vi "Main.vi"(10 "JQMHStartup":refnum<class "ModuleStartup.lvclass">, 11 "SingleLoopTemplate in":refnum<class "SingleLoopTemplate.lvclass">) -> ()   [LabVIEW 2024, in "SingleLoopTemplate.lvclass"]
uses:
  SingleLoopTemplate.lvclass
  RQMHCore/ModuleCore/Module.lvclass/Module.ctl
  RQMHCore/ActionStack/Stack/Stack.lvclass/Stack.ctl
  SingleLoopTemplate.lvclass/SingleLoopTemplate.ctl
  C:/Git/JA/JQMH/RQMHCore/ModuleCore/Module.lvclass
  C:/Git/JA/JQMH/ModuleTemplates/SingleLoopTemplate/SingleLoopTemplate.lvclass
  RQMHCore/ModuleCore/Module.lvclass
  RQMHCore/Startup/ModuleStartup.lvclass
  RQMHCore/ModuleCore/Reply.ctl
  <vilib>/Utility/miscctls.llb/LVPointTypeDef.ctl
  RQMHCore/ModuleCore/InitialiseReplyArgs.ctl
  Do Something ReplyArgs.ctl
  RQMHCore/ActionStack/Stack/Stack.lvclass
  RQMHCore/ActionStack/Stack/StackFromSingleWithPayload.vi
  RQMHCore/ActionStack/Stack/InitFromString.vi
  RQMHCore/ActionStack/Stack/AppendStacks.vi
panel:
  out "error out":errorcluster
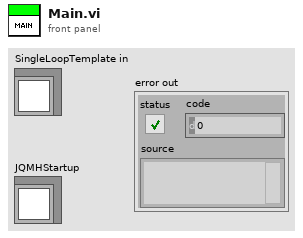
[diagram p1: front panel]
types:
  T1 = typedef "SingleLoopTemplate.lvclass/Request Events--cluster.ctl" = cluster{"Do Something":refnum<user-event>}
  T2 = cluster{"StandardRequests":refnum<event-registration>, "Event Registration Refnum":refnum<event-registration>}
  T3 = cluster{"Module":refnum<class "SingleLoopTemplate.lvclass">, "Args":string}
  T4 = typedef "Module.lvclass/Reply.ctl" = cluster{"Expects Reply":bool, "Reply":refnum<notifier>}
  T5 = enum32{"Invalid", "Standard", "Closed", "Hidden", "Minimized", "Maximized"}
  T6 = typedef "Module.lvclass/InitialiseReplyArgs.ctl" = cluster{"Did Init?":bool}
  T7 = typedef "LVPointTypeDef.ctl" = cluster{"Horizontal":i16, "Vertical":i16}
  T8 = typedef "SingleLoopTemplate.lvclass/Do Something ReplyArgs.ctl" = cluster{"Value":dbl}
  T9 = typedef "JQMHModule.lvclass/Show Front Panel--Args.ctl" = variant
  T10 = typedef "JQMHModule.lvclass/Show Block Diagram.ctl" = bool
  T11 = typedef "JQMHModule.lvclass/Reply.ctl" = cluster{"Expects Reply":bool, "Reply":refnum<notifier>}
  T12 = typedef "SingleLoopTemplate.lvclass/Do Something Args.ctl" = cluster{"Msg":string}
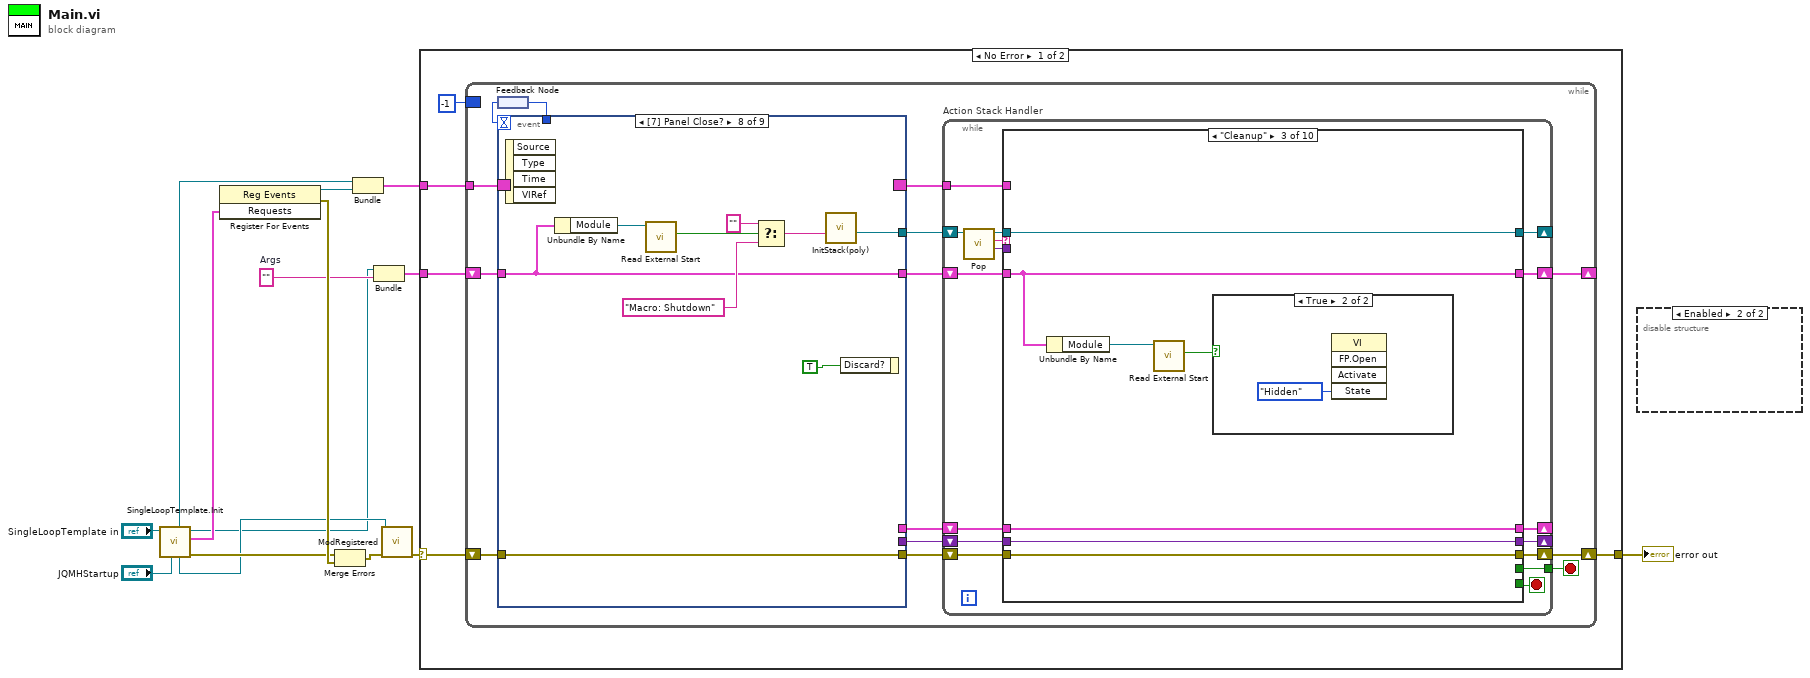
[diagram p0: block diagram]
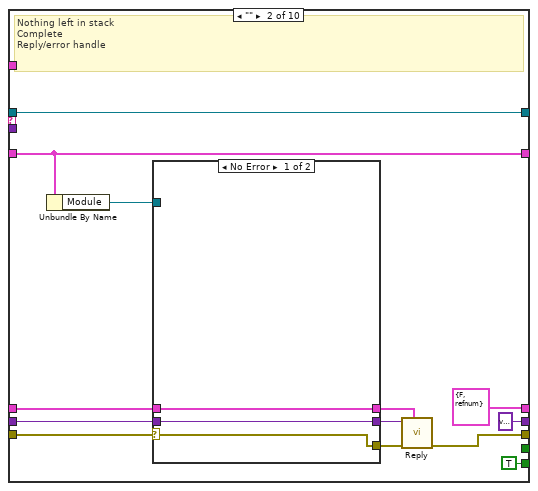
[diagram p3: hidden frame]
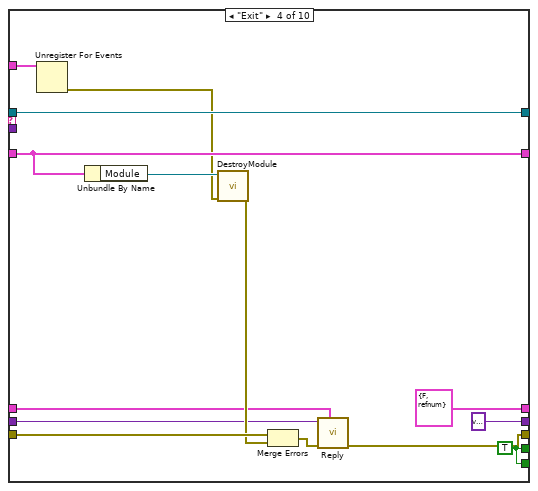
[diagram p6: hidden frame]
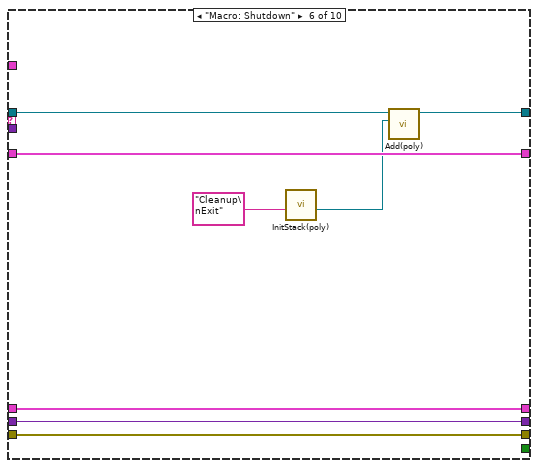
[diagram p8: hidden frame]
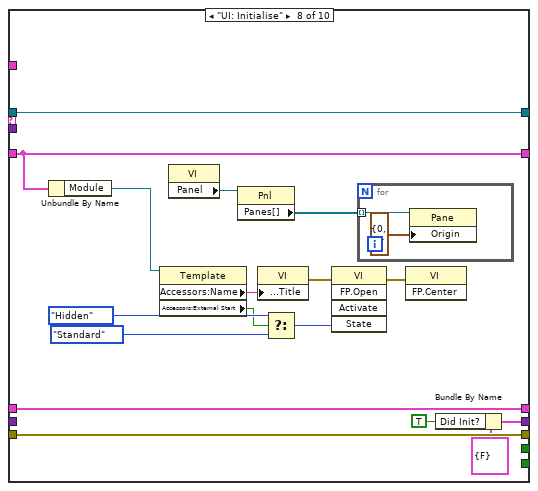
[diagram p10: hidden frame]
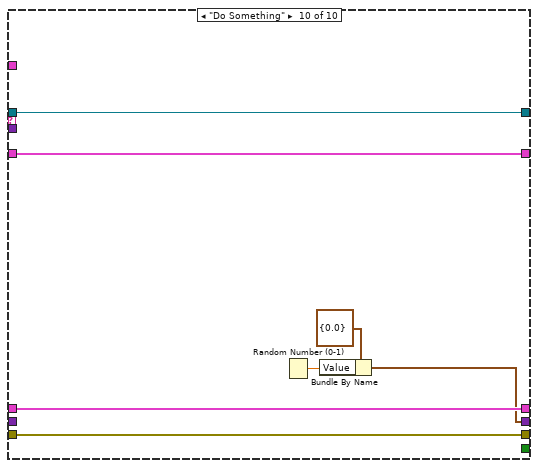
[diagram p12: hidden frame]
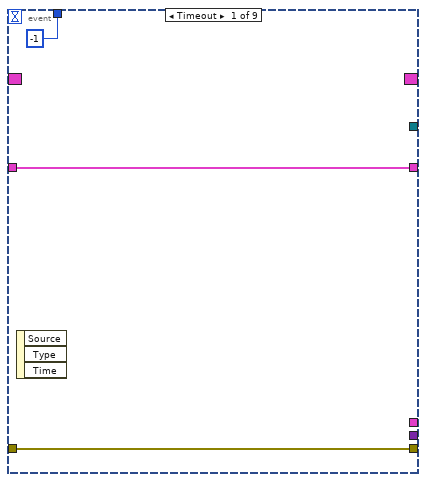
[diagram p13: hidden frame]
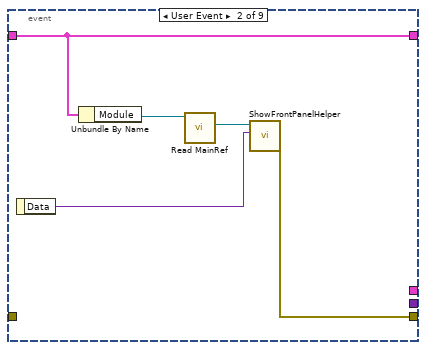
[diagram p14: hidden frame]
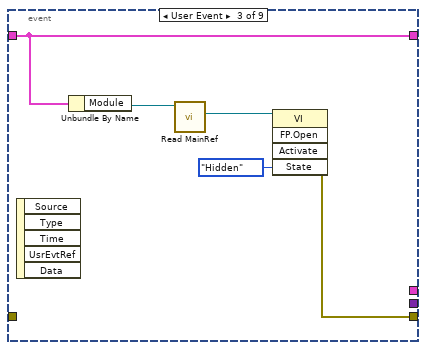
[diagram p15: hidden frame]
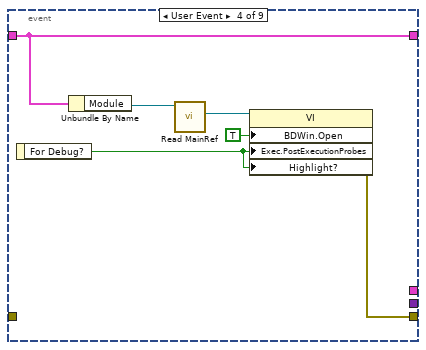
[diagram p16: hidden frame]
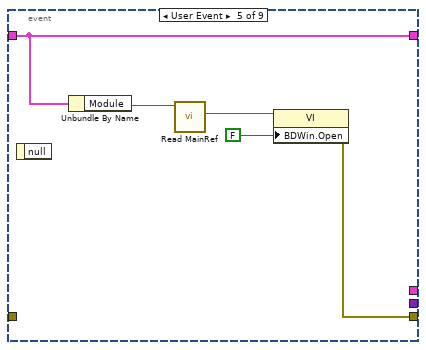
[diagram p17: hidden frame]
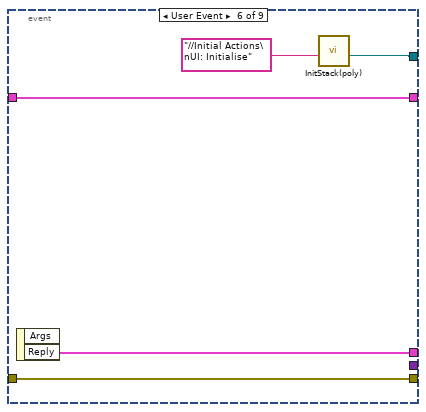
[diagram p18: hidden frame]
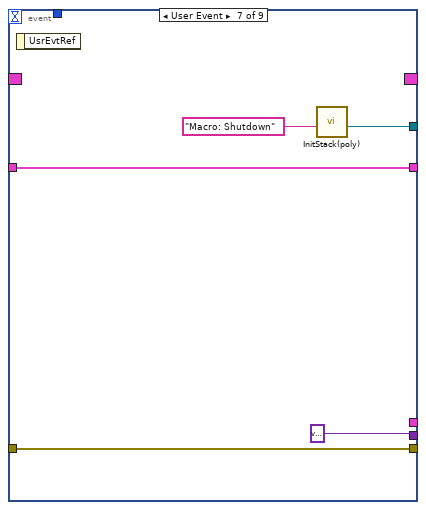
[diagram p19: hidden frame]
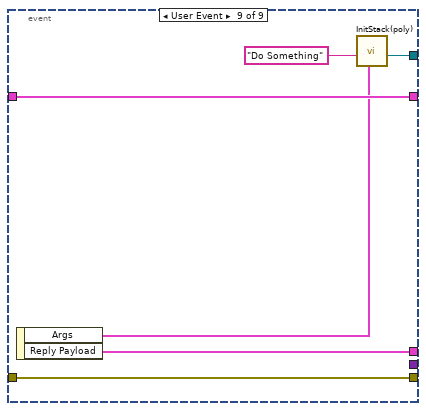
[diagram p20: hidden frame]
diagram:
  w3 = ""  # Args
  n1 = call "SingleLoopTemplate.Init.vi"("JQMHStartup in"="JQMHStartup", "SingleLoopTemplate in"="SingleLoopTemplate in") -> ("error out"=w11:errorcluster, "Requests"=w6:T1, "Module"=w1:refnum<class "SingleLoopTemplate.lvclass">, "JQMHStartup out"=w10:refnum<class "ModuleStartup.lvclass">, "StandardRequests"=w2:refnum<event-registration>)  [unwired: 3 in, 2 out]
  n2 = register-events(w6) -> (reference out=w7:refnum<event-registration>, error out=w15:errorcluster)  [unwired: 2 in]
  n3 = Merge Errors(w11, w15) -> (w8:errorcluster)
  n4 = Bundle("StandardRequests"=w2, "Event Registration Refnum"=w7) -> (w4:T2)  [unwired: 1 in]
  n5 = Bundle("Module"=w1, "Args"=w3) -> (w5:T3)  [unwired: 1 in]
  n6 = call "ModRegistered.vi"("error in (no error)"=w8, "JQMHStartup in"=w10) -> ("error out"=w9:errorcluster)  [unwired: 9 in]
  n7 = case "RQMH_MAIN" shown="No Error" w9 {
    selector: w9 -> [w19 w198]
    tunnel: w4 -> [w17 w197]
    tunnel: [w20 w198] -> w13
    tunnel: w5 -> [w18 w196]
    frame No Error {
      n8 = while {
        shift-right: [w27] -> w20
        shift-left: w19 -> [w34]
        shift-right: [w29] -> _
        shift-left: w18 -> [w30]
        tunnel: w17 -> [w23]
        border: -1 -> [_]
        stop <- w26 stop-if-true
        n9 = feedback #1() -> (w22:i32)
        n10 = event "RQMH_EVENT_MAIN" shown="[7] Panel Close?" {
          selector: w23 -> [_ _ _ _ _ _ _ _ _]
          dyn-events: [_ _ _ _ _ _ _ _ _] -> w33
          timeout: w22 -> [_ _ _ _ _ _ _ _ _]
          tunnel: w34 -> [w148 _ _ _ _ w174 w179 w188 w194]
          tunnel: [w148 w150 w154 w159 w165 w174 w179 w188 w194] -> w28
          tunnel: [_ _ _ _ _ w170 w175 w181 w189] -> w32
          tunnel: w30 -> [w147 w153 w156 w163 w168 w173 w177 w180 w192]
          tunnel: [w147 w153 w156 w163 w168 w173 w177 w180 w192] -> w31
          tunnel: [_ _ _ _ _ w172 _ _ w190] -> w25
          tunnel: [_ _ _ _ _ _ variant _ _] -> w24
          tunnel: [-1 _ _ _ _ _ _ _ _] -> w21
          event Timeout {
            n11 = event-data() -> ()  [unwired: 1 in, 3 out]
          }
          event User Event {
            n12 = event-data() -> ("Data"=w149:T9)  [unwired: 1 in]
            n13 = Unbundle By Name(w153) -> ("Module"=w152:refnum<class "SingleLoopTemplate.lvclass">)
            n14 = call "Read MainRef.vi"("RQMHModule in"=w152) -> ("MainRef"=w151:refnum<vi>)  [unwired: 8 in, 2 out]
            n15 = call "ShowFrontPanelHelper.vi"("Data"=w149, "VI in"=w151) -> ("error out"=w150:errorcluster)  [unwired: 9 in]
          }
          event User Event {
            n16 = event-data() -> ()  [unwired: 1 in, 5 out]
            n17 = Unbundle By Name(w156) -> ("Module"=w157:refnum<class "SingleLoopTemplate.lvclass">)
            n18 = call "Read MainRef.vi"("RQMHModule in"=w157) -> ("MainRef"=w155:refnum<vi>)  [unwired: 8 in, 2 out]
            n19 = invoke class="VI" method="FP.Open"(reference=w155, "State"=T5."Hidden") -> (error out=w154:errorcluster)  [unwired: 3 in, 4 out]
          }
          event User Event {
            n20 = event-data() -> ("For Debug?"=w160:T10)  [unwired: 1 in]
            n21 = Unbundle By Name(w163) -> ("Module"=w164:refnum<class "SingleLoopTemplate.lvclass">)
            n22 = call "Read MainRef.vi"("RQMHModule in"=w164) -> ("MainRef"=w161:refnum<vi>)  [unwired: 8 in, 2 out]
            n23 = property class="VI"(reference=w161, "BDWin.Open"=TRUE ("Block Diagram Window:Open"), "Exec.PostExecutionProbes"=w160, "Highlight?"=w160) -> (error out=w159:errorcluster)  [unwired: 1 in, 1 out]
          }
          event User Event {
            n24 = event-data() -> ()  [unwired: 1 in, 1 out]
            n25 = Unbundle By Name(w168) -> ("Module"=w169:refnum<class "SingleLoopTemplate.lvclass">)
            n26 = call "Read MainRef.vi"("RQMHModule in"=w169) -> ("MainRef"=w166:refnum<vi>)  [unwired: 8 in, 2 out]
            n27 = property class="VI"(reference=w166, "BDWin.Open"=FALSE ("Block Diagram Window:Open")) -> (error out=w165:errorcluster)  [unwired: 1 in, 1 out]
          }
          event User Event {
            n28 = event-data() -> ("Reply"=w172:T11)  [unwired: 1 in, 1 out]
            n29 = call-poly "InitStack(poly).vi"("ActionStack String"="//Initial Actions\nUI: Initialise") -> ("ActionStack out"=w170:refnum<class "Stack.lvclass">)  [unwired: 10 in]
          }
          event User Event {
            (unwired) errorcluster {"status"=FALSE, "code"=0, "source"=""} ("error out")
            (unwired) TRUE
            n30 = event-data() -> ()  [unwired: 1 in, 1 out]
            n31 = call-poly "InitStack(poly).vi"("Action"="Macro: Shutdown") -> ("Stack out"=w175:refnum<class "Stack.lvclass">)  [unwired: 10 in]
          }
          event Panel Close? {
            n32 = event-data() -> ()  [unwired: 1 in, 4 out]
            n33 = Unbundle By Name(w180) -> ("Module"=w186:refnum<class "SingleLoopTemplate.lvclass">)
            n34 = call "Read External Start.vi"("JQMHModule in"=w186) -> ("External Start?"=w185:bool)  [unwired: 8 in, 2 out]
            n35 = Select(t="", s=w185, f="Macro: Shutdown" ("Action")) -> (s? t:f=w182:string)
            n36 = call-poly "InitStack(poly).vi"("Action"=w182) -> ("Stack out"=w181:refnum<class "Stack.lvclass">)  [unwired: 10 in]
            n37 = event-data("Discard?"=TRUE) -> ()  [unwired: 1 in, 1 out]
          }
          event User Event {
            n38 = event-data() -> ("Args"=w191:T12, "Reply Payload"=w190:T4)  [unwired: 1 in]
            n39 = call-poly "InitStack(poly).vi"("Payload"=w191, "Action"="Do Something" ("Message")) -> ("Stack out"=w189:refnum<class "Stack.lvclass">)  [unwired: 9 in]
          }
        }
        n40 = feedback-in #1(w21) -> ()
        n41 = while "Action Stack Handler" {
          shift-right: [w50] -> _
          shift-left: w32 -> [w42]
          shift-right: [w47] -> w27
          shift-left: w28 -> [w48]
          tunnel: w33 -> [w46]
          shift-right: [w44] -> w29
          shift-left: w31 -> [w45]
          tunnel: [w43] -> w26
          shift-right: [w37] -> _
          shift-left: w25 -> [w38]
          shift-right: [w36] -> _
          shift-left: w24 -> [w35]
          stop <- w49 stop-if-true
          n42 = call "Pop.vi"("Stack in"=w42) -> ("Popped Payload"=w39:variant, "Popped Action"=w40:string, "Stack out"=w41:refnum<class "Stack.lvclass">)  [unwired: 8 in]
          n43 = case shown="\"Cleanup\"" w40 {
            tunnel: w41 -> [w55 w68 w81 w96 w101 w103 w114 w131 w138 w145]
            tunnel: [w55 w68 w81 w96 w101 w106 w114 w131 w138 w145] -> w50
            tunnel: w39 -> [_ _ _ _ _ _ _ _ _ _]
            tunnel: [_ TRUE ("Boolean") _ w94 _ _ _ _ _ _] -> w49
            tunnel: w48 -> [w51 w66 w80 w88 w99 w108 w113 w130 w137 w144]
            tunnel: [w51 w61 w80 w83 w99 w108 w113 w130 w137 w144] -> w47
            tunnel: w46 -> [_ _ _ w95 _ _ _ _ _ _]
            tunnel: w45 -> [w54 w65 w75 w90 w100 w109 w112 w127 w136 w143]
            tunnel: [w54 w65 w75 w90 w100 w109 w112 w127 w136 w143] -> w44
            tunnel: [_ _ _ w94 _ _ _ _ _ _] -> w43
            tunnel: w38 -> [w53 w62 w79 w84 w98 w105 w111 w129 w135 w142]
            tunnel: [w53 T4 {"Expects Reply"=FALSE, "Reply"=refnum} ("Reply Payload") w79 T4 {"Expects Reply"=FALSE, "Reply"=refnum} ("Reply Payload") w98 w105 w111 w129 w135 w142] -> w37
            tunnel: [w52 variant ("Variant") w78 variant ("Variant") w97 w104 w110 w122 w134 w139] -> w36
            tunnel: w35 -> [w52 w57 w78 w85 w97 w104 w110 _ w134 _]
            frame Default {
              # "#TODO Add Error Handling"
            }
            frame "" {
              # "Nothing left in stack\nComplete\nReply/error handle"
              n44 = Unbundle By Name(w65) -> ("Module"=w64:refnum<class "SingleLoopTemplate.lvclass">)
              n45 = case shown="No Error" w66 {
                selector: w66 -> [w69 w73]
                tunnel: [w71 w74] -> w63
                tunnel: w62 -> [w71 w74]
                tunnel: [w70 w72] -> w58
                tunnel: w57 -> [w70 w72]
                tunnel: w64 -> [_ _]
                tunnel: [w69 w73] -> w56
                frame No Error {
                }
                frame Error {
                }
              }
              n46 = call "Reply.vi"("Reply"=w63, "error in (no error)"=w56, "ReplyPayload"=w58) -> ("error out"=w61:errorcluster)  [unwired: 8 in]
            }
            frame "Cleanup" {
              n47 = Unbundle By Name(w75) -> ("Module"=w77:refnum<class "SingleLoopTemplate.lvclass">)
              n48 = call "Read External Start.vi"("JQMHModule in"=w77) -> ("External Start?"=w76:bool)  [unwired: 8 in, 2 out]
              n49 = case shown="True" w76 {
                frame False {
                }
                frame True {
                  n50 = invoke class="VI" method="FP.Open"("State"=T5."Hidden") -> ()  [unwired: 4 in, 5 out]
                }
              }
            }
            frame "Exit" {
              w94 = TRUE
              n51 = Unregister For Events(event registration refnum=w95) -> (error out=w89:errorcluster)  [unwired: 1 in]
              n52 = Unbundle By Name(w90) -> ("Module"=w91:refnum<class "SingleLoopTemplate.lvclass">)
              n53 = call "DestroyModule.vi"("error in (no error)"=w89, "JQMHModule in"=w91) -> ("error out"=w87:errorcluster)  [unwired: 9 in]
              n54 = Merge Errors(w88, w87) -> (w86:errorcluster)
              n55 = call "Reply.vi"("Reply"=w84, "error in (no error)"=w86, "ReplyPayload"=w85) -> ("error out"=w83:errorcluster)  [unwired: 8 in]
            }
            frame "---------- Macros ----------" {
            }
            frame "Macro: Shutdown" {
              n56 = call-poly "InitStack(poly).vi"("ActionStack String"="Cleanup\nExit") -> ("ActionStack out"=w102:refnum<class "Stack.lvclass">)  [unwired: 10 in]
              n57 = call-poly "Add(poly).vi"("Second"=w102, "First"=w103) -> ("First"=w106:refnum<class "Stack.lvclass">)  [unwired: 9 in]
            }
            frame "---------- UI ----------" {
              # "Add module specific commands"
            }
            frame "UI: Initialise" {
              n58 = Unbundle By Name(w127) -> ("Module"=w126:refnum<class "SingleLoopTemplate.lvclass">)
              n59 = property class="Template"(reference=w126) -> ("Accessors:Name"=w117:string, "Accessors:External Start"=w116:bool)  [unwired: 1 in, 2 out]
              n60 = property on="Property Node" class="VI"() -> ("Panel"=w119:refnum<vi>)  [unwired: 2 in, 2 out]
              n61 = property on="Property Node" class="Pnl"(reference=w119) -> ("Panes[]"=w118:refnum<vi>[])  [unwired: 1 in, 2 out]
              n62 = property on="Property Node" class="VI"("Front Panel.Title"=w117) -> (error out=w121:errorcluster)  [unwired: 2 in, 1 out]
              n63 = Select(t=T5."Hidden" ("State"), s=w116, f=T5."Standard" ("State")) -> (s? t:f=w115:T5)
              n64 = invoke on="Invoke Node" class="VI" method="FP.Open"(error in=w121, "State"=w115) -> (error out=w120:errorcluster)  [unwired: 3 in, 4 out]
              n65 = for {
                tunnel: w118 -> [w132] mode=indexing
                n66 = property on="Property Node" class="Pane"(reference=w132, "Origin"=T7 {"Horizontal"=0, "Vertical"=0}) -> ()  [unwired: 1 in, 2 out]
              }
              n67 = invoke on="Invoke Node" class="VI" method="FP.Center"(error in=w120) -> ()  [unwired: 2 in, 3 out]
              n68 = Bundle By Name(cluster=T6 {"Did Init?"=FALSE} ("Args"), "Did Init?"=TRUE) -> (w122:T6)
            }
            frame "---------- Actions ----------" {
              # "Add module specific commands"
            }
            frame "Do Something" {
              n69 = Random Number (0-1)() -> (number: 0 to 1=w141:dbl)
              n70 = Bundle By Name(cluster=T8 {"Value"=0.0} ("ReplyArgs"), "Value"=w141) -> (w139:T8)
            }
          }
        }
      }
    }
    frame Error {
      n71 = Unregister For Events(event registration refnum=w197) -> ()  [unwired: 1 in, 1 out]
      n72 = Unbundle(w196) -> ("Module"=w195:refnum<class "SingleLoopTemplate.lvclass">)  [unwired: 1 out]
      n73 = call "DestroyModule.vi"("JQMHModule in"=w195) -> ()  [unwired: 10 in, 1 out]
    }
  }
  "error out" <- w13
  n74 = disable-structure shown="Enabled" {
    frame Disabled {
    }
    frame Enabled {
    }
  }
